vi "niRFUtil CONV 1 Ohm Voltage to 1 Ohm Watt (complex wfm).vi"(7 "Complex Waveform (V)":T3 {"y" format="%.2f"; "dx" format="%^.2e"; "x0" format="%^.2e"}) -> (8 "Real Waveform (W)":T1 {"y" min=0 max=127 format="%.2f"; "dx" format="%^.2e"; "x0" format="%^.2e"})   [LabVIEW 2015, in "niRFUtil.lvlib"]
doc: "(c) Copyright 2006, National Instruments, Inc. This VI may not be duplicated, sold, or distributed without written consent from National Instruments."
uses:
  niRFUtil.lvlib
  Includes/niRFUtil INC Complex Waveform.ctl
  Includes/niRFUtil INC Complex Array.ctl
  Includes/niRFUtil INC Real Waveform.ctl
  Includes/niRFUtil INC Real Array.ctl
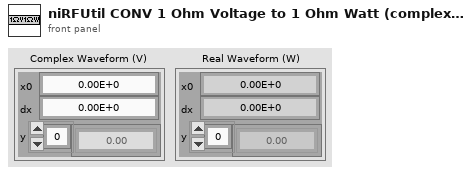
[diagram p1: front panel]
types:
  T1 = typedef "niRFUtil.lvlib/niRFUtil INC Real Waveform.ctl" = cluster{"x0":dbl, "dx":dbl, "y":T2}
  T2 = typedef "niRFUtil.lvlib/niRFUtil INC Real Array.ctl" = sgl[]
  T3 = typedef "niRFUtil.lvlib/niRFUtil INC Complex Waveform.ctl" = cluster{"x0":dbl, "dx":dbl, "y":T4}
  T4 = typedef "niRFUtil.lvlib/niRFUtil INC Complex Array.ctl" = csg[]
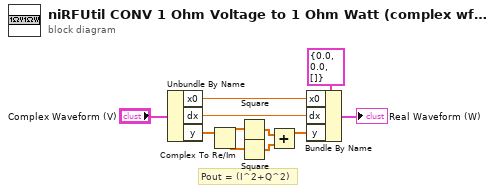
[diagram p0: block diagram]
diagram:
  # "Pout = (I^2+Q^2)"
  n1 = Unbundle By Name("Complex Waveform (V)") -> ("x0"=w2:dbl, "dx"=w1:dbl, "y"=w7:T4)
  n2 = Complex To Re/Im(x + iy=w7) -> (x=w6:sgl[], y=w5:sgl[])
  n3 = Square(x=w6) -> (x^2=w4:sgl[])
  n4 = Square(x=w5) -> (x^2=w3:sgl[])
  n5 = Add(x=w4, y=w3) -> (x+y=w8:sgl[])
  n6 = Bundle By Name(cluster=T1 {"x0"=0.0, "dx"=0.0, "y"=[]} ("Real Waveform (W)"), "x0"=w2, "dx"=w1, "y"=w8) -> (→"Real Waveform (W)":T1)
